vi "Construct Rx.vi"(7 "timing channel offset (-1)":i64=-1, 8 "error in":errorcluster, 10 "Rx hardware channels in":T2[](array[typedef]) {"labels settings for RT"."Label Timestamp Channel Data Reference" format="%.0x"; "labels settings for RT"."Word Initial Raw Value" format="%032.0f"; "labels settings for RT"."Label Disable/Trigger Channel Reference" format="%.0x"; "labels settings for RT"."parameter driver data"."Tx parameter refs" format="%.0x"; "labels settings for RT"."SDI" format="%02b"; "labels settings for RT"."label" format="%.0o"}, 11 "custom device ref in":T1=18446744073709551615 format="%.0x") -> (0 "error out":errorcluster, 2 "Rx Execution Unit out":refnum<class "Rx Execution Unit.lvclass">, 3 "custom device ref out":T1=18446744073709551615 format="%.0x")   [LabVIEW 2020, in "AIM ARINC 429 Engine.lvlib" / "Implementation.lvlib" / "Rx Execution Unit.lvclass"]
doc: "Constructs a new Rx Execution Unit object."
uses:
  Rx Execution Unit.lvclass
  Execution Unit/Execution Unit.lvclass
  Execution Unit Factory/Execution Unit Factory.lvclass
  C:/Users/nitest/Desktop/Git 2020/niveristand-aim-arinc429-custom-device/Source/Custom Device Support/Engine/Implementation/Execution Unit/Execution Unit.lvclass
  Shared/Label.ctl
  <vilib>/NI/NI VeriStand Encoding and Decoding/Encoding.ctl
  <vilib>/NI/NI VeriStand Encoding and Decoding/Encoding and Decoding.lvlib
  Shared/Parameter Definition.ctl
  <vilib>/NI VeriStand/Custom Device API/Custom Device Item Ref.ctl
  <vilib>/NI VeriStand/Custom Device API/Custom Device API.lvlib
  Shared/RT Parameters.ctl
  Shared/Transfer Type.ctl
  <vilib>/NI VeriStand/Custom Device API/Data Reference.ctl
  Shared/RT Label Settings.ctl
  Shared/RT Hardware Channel Settings.ctl
  Shared/Transfer Speed.ctl
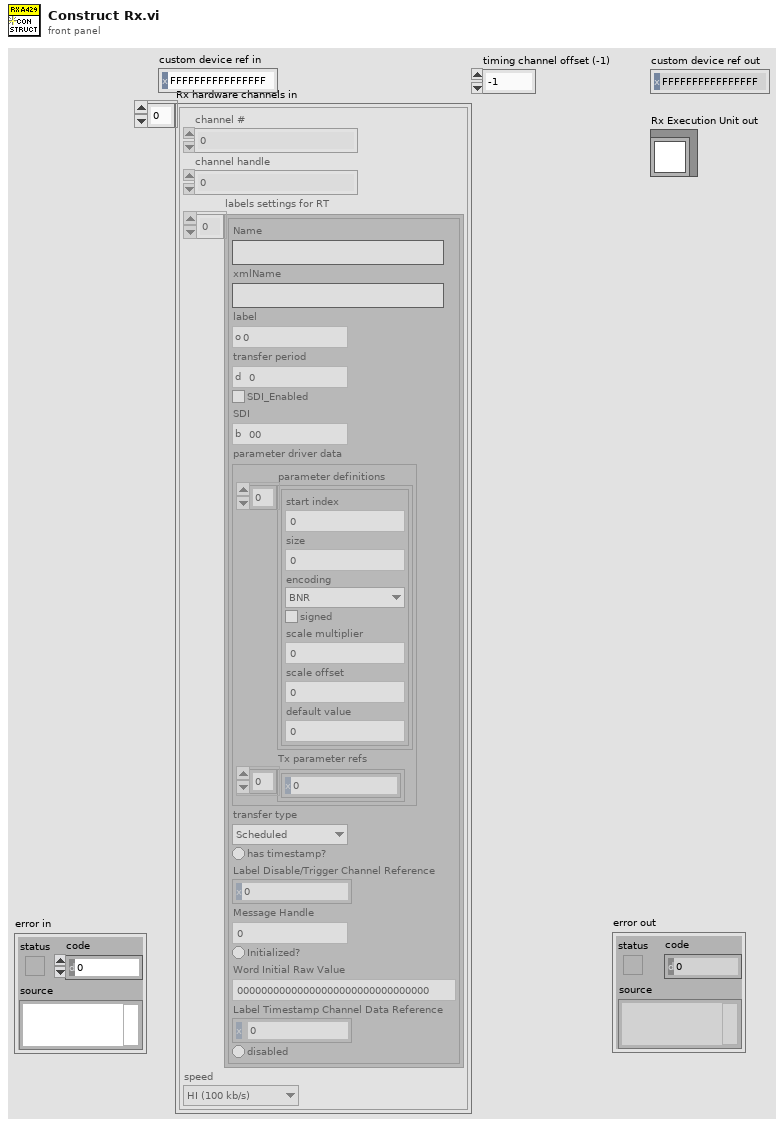
[diagram p1: front panel]
types:
  T1 = typedef "Custom Device API.lvlib/Custom Device Item Ref.ctl" = u64
  T2 = typedef "RT Hardware Channel Settings.ctl" = cluster{"channel #":u16, "channel handle":u64, "labels settings for RT":T3[], "speed":T10}
  T3 = typedef "RT Label Settings.ctl" = cluster{"Name":string, "xmlName":string, "label":T4, "transfer period":u32, "SDI_Enabled":bool, "SDI":u8, "parameter driver data":T5, "transfer type":T8, "has timestamp?":bool, "Label Disable/Trigger Channel Reference":T1, "Message Handle":u64, "Initialized?":bool, "Word Initial Raw Value":u32, "Label Timestamp Channel Data Reference":T9, "disabled":bool}
  T4 = typedef "Label.ctl" = u8
  T5 = typedef "RT Parameters.ctl" = cluster{"parameter definitions":T6[], "Tx parameter refs":T1[]}
  T6 = typedef "Parameter Definition.ctl" = cluster{"start index":i32, "size":i32, "encoding":T7, "signed":bool, "scale multiplier":dbl, "scale offset":dbl, "default value":dbl}
  T7 = typedef "Encoding and Decoding.lvlib/Encoding.ctl" = enum16{"BNR", "BCD", "Discrete"}
  T8 = typedef "Transfer Type.ctl" = enum16{"Scheduled", "Acyclic", "Block", "Strobe"}
  T9 = typedef "Custom Device API.lvlib/Data Reference.ctl" = i32
  T10 = typedef "Transfer Speed.ctl" = enum16{"LO (12.5 kb/s)", "HI (100 kb/s)"}
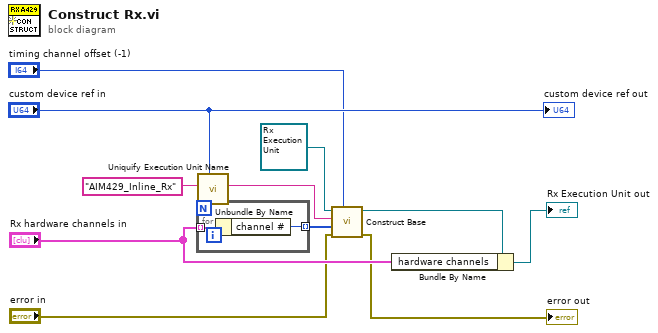
[diagram p0: block diagram]
diagram:
  n1 = for {
    tunnel: "Rx hardware channels in" -> [w13] mode=indexing
    tunnel: [w12] -> w10 mode=indexing
    n2 = Unbundle By Name(w13) -> ("channel #"=w12:u16)
  }
  n3 = call "Uniquify Execution Unit Name.vi"("custom device ref"="custom device ref in", "execution unit name"="AIM429_Inline_Rx" ("identifier in")) -> ("execution unit name out"=w3:string)  [unwired: 9 in]
  n4 = call "Construct Base.vi"("timing channel offset (-1)"="timing channel offset (-1)", "error in (no error)"="error in", "channels"=w10, "identifier in"=w3, "Execution Unit in (default object)"=refnum<class "Rx Execution Unit.lvclass"> refnum ("Rx Execution Unit in")) -> ("error out"=→"error out":errorcluster, "Execution Unit out"=w9:refnum<class "Rx Execution Unit.lvclass">)  [unwired: 5 in]
  n5 = Bundle By Name(cluster=w9, "hardware channels"="Rx hardware channels in") -> (→"Rx Execution Unit out":refnum<class "Rx Execution Unit.lvclass">)
  "custom device ref out" <- "custom device ref in"
